vi "Get or Init Domain Class.vi"(7 "target Domain":refnum<class "NI_Domain.lvclass">, 8 "error in (no error)":errorcluster, 11 "PDE out":refnum<class "NI_PDE.lvclass">) -> (0 "error out":errorcluster, 2 "Domain out":refnum<class "NI_Domain.lvclass">, 3 "PDE in":refnum<class "NI_PDE.lvclass">)   [LabVIEW 2020, in "NI_PDE.lvlib" / "NI_PDE.lvclass"]
uses:
  <vilib>/gmath/pde.llb/PDEClass/NI_PDE.lvclass
  <vilib>/gmath/pde.llb/DomainClass/NI_Domain.lvclass
  <vilib>/gmath/pde.llb/DomainClass/Class Type.ctl
  <vilib>/gmath/pde.llb/Common/PDE_Error.ctl
  <vilib>/gmath/NI_PDE.lvlib
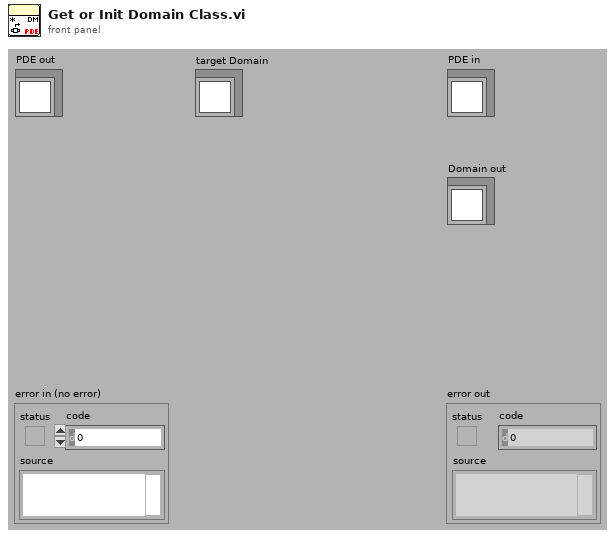
[diagram p1: front panel]
types:
  T1 = typedef "NI_PDE.lvlib/PDE_Error.ctl" = enum16{"No Error", "k is zero", "End point <= start point", "# of time steps < 2", "# of spatial points < 3", "# of grid < 1 for FEM", "# of boundary < 3 for FEM", "Incompatible RHS size", "Incompatible BC size", "Incompatible IC size", "PDE class conflict", "RHS class conflict", "Domain class conflict", "BC class conflict", "IC class conflict"}
  T2 = typedef "NI_PDE.lvlib/NI_Domain.lvclass/Class Type.ctl" = i32
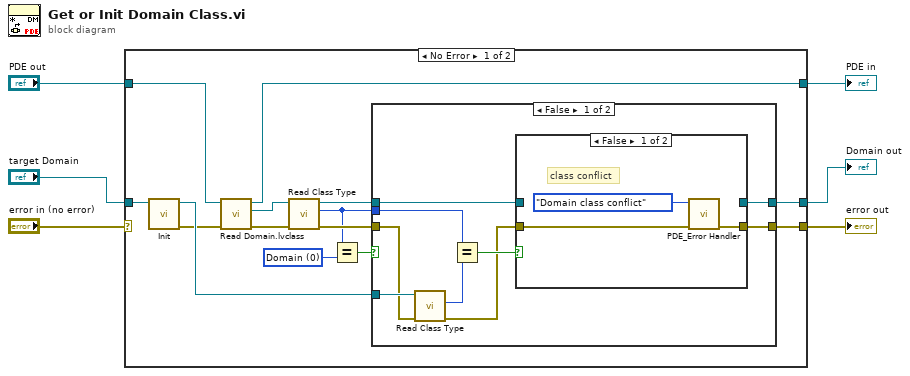
[diagram p0: block diagram]
diagram:
  n1 = case shown="No Error" "error in (no error)" {
    selector: "error in (no error)" -> [_ w39]
    tunnel: "PDE out" -> [w20 w37]
    tunnel: [w13 w38] -> w5
    tunnel: [w12 w39] -> w4
    tunnel: [w11 w37] -> w3
    tunnel: "target Domain" -> [w9 w38]
    frame No Error {
      w10 = T2 0 items=["Domain"=0, "Domain_Steady"=100, "Domain_Steady_2D_Rect"=121, "Domain_Steady_2D_Polygon"=122, "Domain_Evolut"=200, "Domain_Evolut_1D"=210, "Domain_Evolut_2D_Rect"=221] ("domain class type")
      n2 = call-dynamic "Init.vi"("Domain"=w9) -> ("error out"=w7:errorcluster, "initialized Domain"=w8:refnum<class "NI_Domain.lvclass">)  [unwired: 1 in, 8 out]
      n3 = call-dynamic "Read Domain.lvclass.vi"("error in (no error)"=w7, "PDE.lvclass in"=w20) -> ("error out"=w18:errorcluster, "Domain.lvclass"=w19:refnum<class "NI_Domain.lvclass">, "PDE.lvclass out"=w11:refnum<class "NI_PDE.lvclass">)  [unwired: 7 out]
      n4 = call-dynamic "Read Class Type.vi"("error in (no error)"=w18, "Domain.lvclass in"=w19) -> ("error out"=w15:errorcluster, "domain class type"=w14:T2, "Domain.lvclass out"=w16:refnum<class "NI_Domain.lvclass">)  [unwired: 7 out]
      n5 = Equal?(x=w14, y=w10) -> (x = y?=w17:bool)
      n6 = case shown="False" w17 {
        tunnel: w16 -> [w28 _]
        tunnel: w15 -> [w22 w36]
        tunnel: [w26 w35] -> w13
        tunnel: w14 -> [w27 _]
        tunnel: [w25 w36] -> w12
        tunnel: w8 -> [w24 w35]
        frame False {
          n7 = call-dynamic "Read Class Type.vi"("error in (no error)"=w22, "Domain.lvclass in"=w24) -> ("error out"=w21:errorcluster, "domain class type"=w23:T2)  [unwired: 8 out]
          n8 = Equal?(x=w27, y=w23) -> (x = y?=w29:bool)
          n9 = case shown="False" w29 {
            tunnel: w21 -> [w31 w33]
            tunnel: w28 -> [_ w34]
            tunnel: [_ w34] -> w26
            tunnel: [w30 w33] -> w25
            frame False {
              # "class conflict"
              n10 = call <vilib>:"PDE_Error Handler.vi"("error in (no error)"=w31, "PDE error"=PDE_Error."Domain class conflict") -> ("error out"=w30:errorcluster)  [unwired: 9 out]
            }
            frame True {
            }
          }
        }
        frame True {
        }
      }
    }
    frame Error {
    }
  }
  "Domain out" <- w5
  "error out" <- w4
  "PDE in" <- w3
